vi "Clear2DListCtrl.vi"(11 "ArrayRef in":refnum<vi>) -> (3 "ArrayRef out":refnum<vi>)   [LabVIEW 2018, in "Library-Ctrl.lvlib"]
uses:
  Library-Ctrl.lvlib
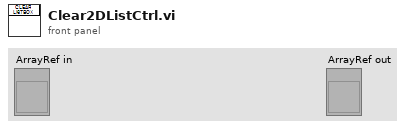
[diagram p1: front panel]
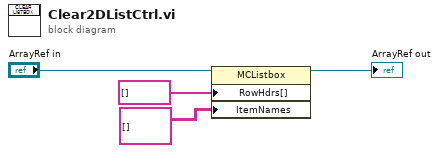
[diagram p0: block diagram]
diagram:
  n1 = property class="MCListbox"(reference="ArrayRef in", "RowHdrs[]"=string[] [] ("행 헤더 문자열[]"), "ItemNames"=string[][] [] ("아이템 이름")) -> (reference out=→"ArrayRef out":refnum<vi>)  [unwired: 1 in, 1 out]
